vi "DashboardLEDStatesFront.vi"(0 "State":string, 2 "Default":string, 3 "Traction":string, 5 "Gear Ready":string) -> (6 "RED":bool, 7 "GREEN":bool, 8 "BLUE":bool)   [LabVIEW 2016]
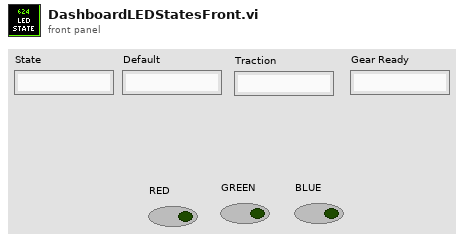
[diagram p1: front panel]
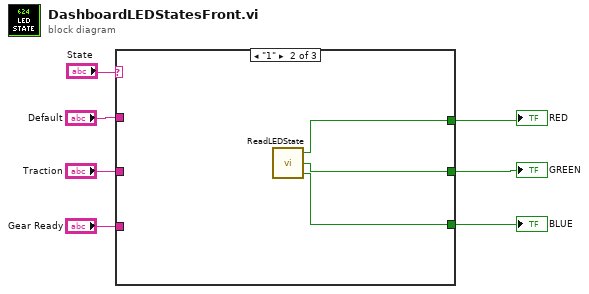
[diagram p0: block diagram]
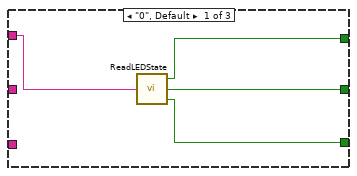
[diagram p2: hidden frame]
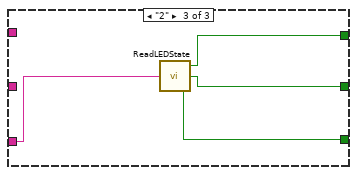
[diagram p3: hidden frame]
diagram:
  n1 = case shown="\"1\"" "State" {
    tunnel: "Default" -> [w11 _ _]
    tunnel: "Traction" -> [_ _ _]
    tunnel: "Gear Ready" -> [_ _ w18]
    tunnel: [w10 w14 w17] -> w4
    tunnel: [w9 w13 w16] -> w3
    tunnel: [w8 w12 w15] -> w2
    frame "0", Default {
      n2 = call "ReadLEDState.vi"("String"=w11) -> ("BLUE"=w8:bool, "GREEN"=w9:bool, "RED"=w10:bool)  [unwired: 2 in]
    }
    frame "1" {
      n3 = call "ReadLEDState.vi"() -> ("BLUE"=w12:bool, "GREEN"=w13:bool, "RED"=w14:bool)  [unwired: 3 in]
    }
    frame "2" {
      n4 = call "ReadLEDState.vi"("String"=w18) -> ("BLUE"=w15:bool, "GREEN"=w16:bool, "RED"=w17:bool)  [unwired: 2 in]
    }
  }
  "RED" <- w4
  "GREEN" <- w3
  "BLUE" <- w2
